vi "SSC DCPower Measure.vi"(0 "DCPower SSC in":T2[](array[typedef]), 5 "Measurement Mode":T1 caption="Measurement Mode (Auto)", 11 "error in":errorcluster) -> (4 "DCPower SSC out":T2[](array[typedef]), 6 "Voltage Measurements (V)":dbl[](array[numeric]) format="%#_6p", 8 "Current Measurements (A)":dbl[](array[numeric]) format="%#_6p", 15 "error out":errorcluster)   [LabVIEW 2020]
doc: "This VI takes a Voltage and Current measurement for each session.\n\nMeasurement Mode is a recommended input. The Auto setting will check the measurement mode for each session and use the appropriate measurement method per session."
uses:
  SSC DCPower.ctl
  Measure/SSC DCPower Measurement Mode.ctl
  <instrlib>/niDCPower/nidcpower.llb/niDCPower Send Software Edge Trigger - Signal.ctl
  Measure/SSC DCPower Debug Global.vi
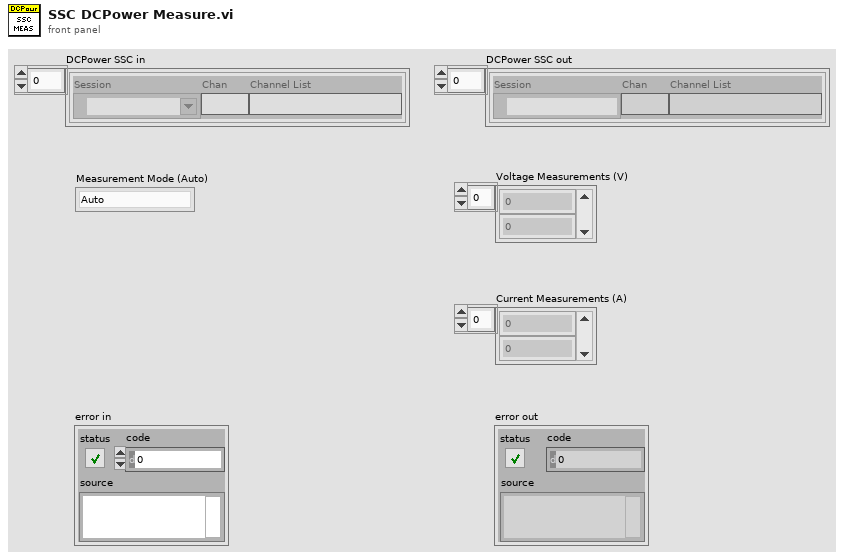
[diagram p1: front panel]
types:
  T1 = typedef "SSC DCPower Measurement Mode.ctl" = enum16{"Auto", "Measure Multiple", "Software Triggers"}
  T2 = typedef "SSC DCPower.ctl" = cluster{"Session":refnum<k15>, "Chan":string, "Channel List":string}
  T3 = typedef "niDCPower Send Software Edge Trigger - Signal.ctl" = i32
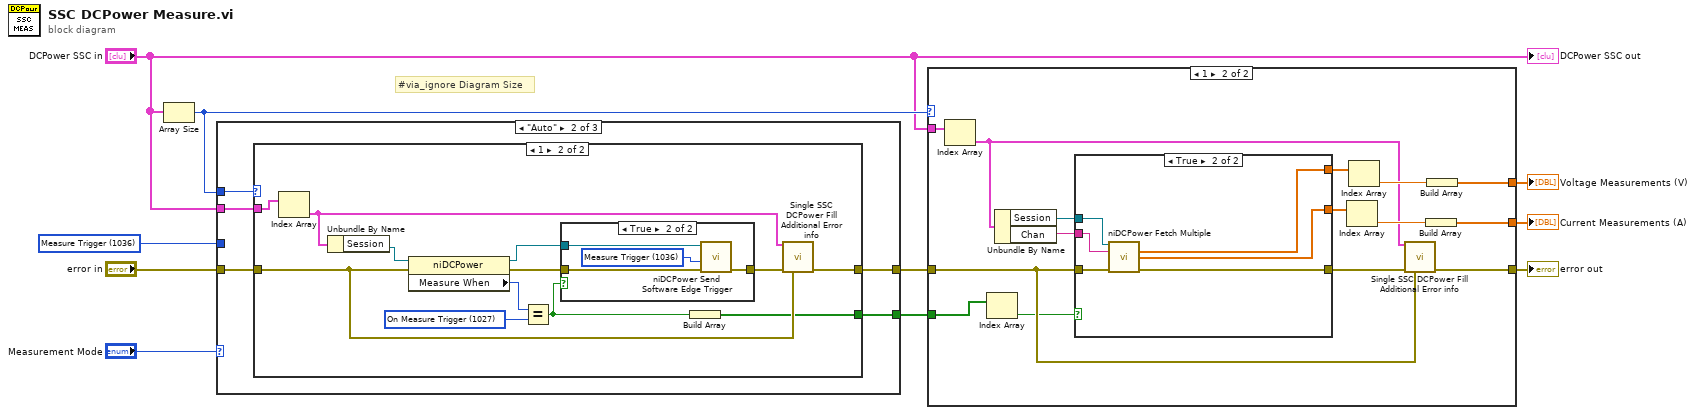
[diagram p0: block diagram]
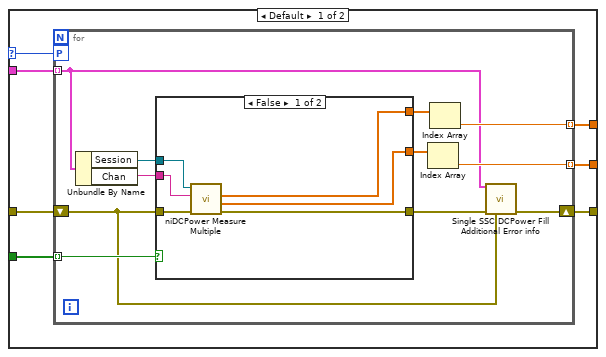
[diagram p2: hidden frame]
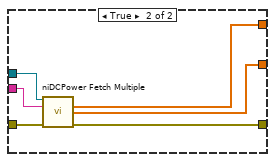
[diagram p3: hidden frame]
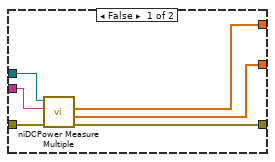
[diagram p4: hidden frame]
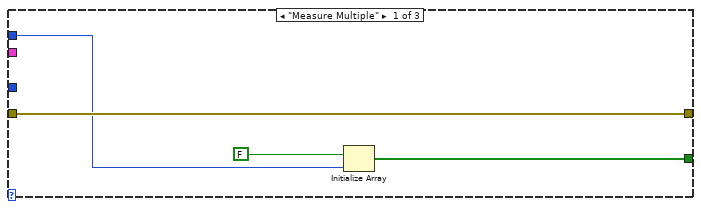
[diagram p5: hidden frame]
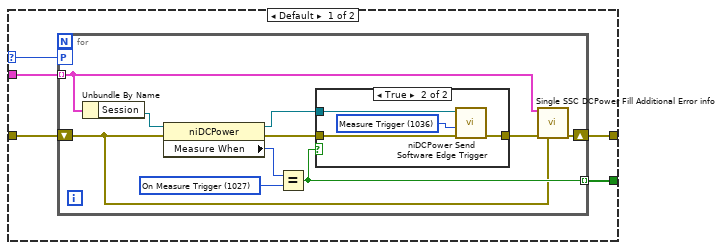
[diagram p6: hidden frame]
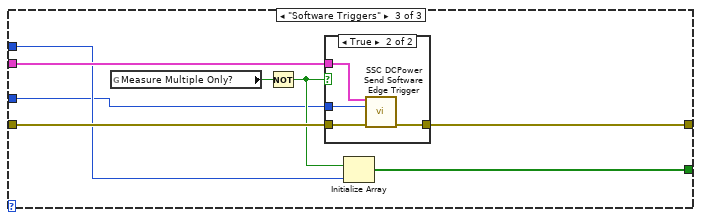
[diagram p9: hidden frame]
diagram:
  w1 = T3 1036 items=["Start Trigger"=1034, "Source Trigger"=1035, "Measure Trigger"=1036, "Sequence Advance Trigger"=1037, "Pulse Trigger"=1053] ("Trigger to Send")
  # "#via_ignore Diagram Size"
  n1 = Array Size(array="DCPower SSC in") -> (size(s)=w7:i32)
  n2 = case shown="\"Auto\"" "Measurement Mode" {
    tunnel: "error in" -> [w14 w19 w64]
    tunnel: [w14 w18 w63] -> w9
    tunnel: w7 -> [w13 w17 w59]
    tunnel: "DCPower SSC in" -> [_ w16 w62]
    tunnel: [w11 w15 w58] -> w3
    tunnel: w1 -> [_ _ w57]
    frame "Measure Multiple" {
      n3 = Initialize Array(FALSE, w13) -> (w11:bool[])
    }
    frame "Auto" {
      n4 = case shown="1" w17 {
        selector: w17 -> [w22 _]
        tunnel: w19 -> [w24 w51]
        tunnel: [w23 w50] -> w18
        tunnel: w16 -> [w21 w49]
        tunnel: [w20 w40] -> w15
        frame Default {
          n5 = for {
            shift-right: [w27] -> w23
            shift-left: w24 -> [w25]
            tunnel: w21 -> [w26] mode=indexing
            workers-P: w22 -> [_]
            tunnel: [w28] -> w20 mode=indexing
            w29 = 1027 items=["Automatically after Source Complete"=1025, "On Demand"=1026, "On Measure Trigger"=1027] ("Measurement:Advanced:Measure When")
            n6 = Unbundle By Name(w26) -> ("Session"=w33:refnum<k15>)
            n7 = property class="niDCPower"(reference=w33, error in=w25) -> (reference out=w31:refnum<k15>, error out=w34:errorcluster, "Measure When"=w30:i32)
            n8 = Equal?(x=w30, y=w29) -> (x = y?=w28:bool)
            n9 = case shown="True" w28 {
              tunnel: w34 -> [w35 w39]
              tunnel: [w35 w38] -> w32
              tunnel: w31 -> [_ w37]
              frame False {
              }
              frame True {
                w36 = T3 1036 items=["Start Trigger"=1034, "Source Trigger"=1035, "Measure Trigger"=1036, "Sequence Advance Trigger"=1037, "Pulse Trigger"=1053] ("signal")
                n10 = call <instrlib>:"niDCPower Send Software Edge Trigger.vi"("error in (no error)"=w39, "signal"=w36, "instrument handle"=w37) -> ("error out"=w38:errorcluster)  [unwired: 7 in, 1 out]
              }
            }
            n11 = call "Single SSC DCPower Fill Additional Error info.vi"("DCPower SSC in"=w26, "error in"=w32, "previous error in"=w25) -> ("error out"=w27:errorcluster)  [unwired: 12 in]
          }
        }
        frame 1 {
          w42 = 1027 items=["Automatically after Source Complete"=1025, "On Demand"=1026, "On Measure Trigger"=1027] ("Measurement:Advanced:Measure When")
          n12 = Index Array(array=w49) -> (element=w41:T2)  [unwired: 1 in]
          n13 = Unbundle By Name(w41) -> ("Session"=w46:refnum<k15>)
          n14 = property class="niDCPower"(reference=w46, error in=w51) -> (reference out=w44:refnum<k15>, error out=w47:errorcluster, "Measure When"=w43:i32)
          n15 = Equal?(x=w43, y=w42) -> (x = y?=w48:bool)
          n16 = case shown="True" w48 {
            tunnel: w47 -> [w52 w56]
            tunnel: [w52 w55] -> w45
            tunnel: w44 -> [_ w54]
            frame False {
            }
            frame True {
              w53 = T3 1036 items=["Start Trigger"=1034, "Source Trigger"=1035, "Measure Trigger"=1036, "Sequence Advance Trigger"=1037, "Pulse Trigger"=1053] ("signal")
              n17 = call <instrlib>:"niDCPower Send Software Edge Trigger.vi"("error in (no error)"=w56, "signal"=w53, "instrument handle"=w54) -> ("error out"=w55:errorcluster)  [unwired: 7 in, 1 out]
            }
          }
          n18 = Build Array(w48) -> (w40:bool[])
          n19 = call "Single SSC DCPower Fill Additional Error info.vi"("DCPower SSC in"=w41, "error in"=w45, "previous error in"=w51) -> ("error out"=w50:errorcluster)  [unwired: 12 in]
        }
      }
    }
    frame "Software Triggers" {
      n20 = global read "SSC DCPower Debug Global.vi" "Measure Multiple Only?"() -> (w61:bool)
      n21 = Not(x=w61) -> (.not. x?=w60:bool)
      n22 = case shown="True" w60 {
        tunnel: w64 -> [w65 w69]
        tunnel: [w65 w68] -> w63
        tunnel: w62 -> [_ w67]
        tunnel: w57 -> [_ w66]
        frame False {
        }
        frame True {
          n23 = call "SSC DCPower Send Software Edge Trigger.vi"("DCPower SSC in"=w67, "Trigger to Send"=w66, "error in"=w69) -> ("error out"=w68:errorcluster)  [unwired: 11 in, 1 out]
        }
      }
      n24 = Initialize Array(w60, w59) -> (w58:bool[])
    }
  }
  n25 = case shown="1" w7 {
    selector: w7 -> [w74 _]
    tunnel: w9 -> [w76 w114]
    tunnel: [w75 w113] -> w8
    tunnel: "DCPower SSC in" -> [w73 w112]
    tunnel: [w72 w101] -> w5
    tunnel: [w71 w100] -> w4
    tunnel: w3 -> [w70 w109]
    frame Default {
      n26 = for {
        shift-right: [w79] -> w75
        shift-left: w76 -> [w77]
        workers-P: w74 -> [_]
        tunnel: w73 -> [w78] mode=indexing
        tunnel: [w82] -> w72 mode=indexing
        tunnel: [w80] -> w71 mode=indexing
        tunnel: w70 -> [w84] mode=indexing
        n27 = Unbundle By Name(w78) -> ("Session"=w86:refnum<k15>, "Chan"=w85:string)
        n28 = case shown="False" w84 {
          tunnel: w77 -> [w93 w99]
          tunnel: [w92 w98] -> w87
          tunnel: w86 -> [w91 w97]
          tunnel: w85 -> [w90 w95]
          tunnel: [w89 w96] -> w83
          tunnel: [w88 w94] -> w81
          frame False {
            n29 = call <instrlib>:"niDCPower Measure Multiple.vi"("error in (no error)"=w93, "channel name"=w90, "instrument handle"=w91) -> ("error out"=w92:errorcluster, "current measurements"=w88:dbl[], "voltage measurements"=w89:dbl[])  [unwired: 5 in, 1 out]
          }
          frame True {
            n30 = call <instrlib>:"niDCPower Fetch Multiple.vi"("instrument handle"=w97, "channel name"=w95, "error in (no error)"=w99) -> ("voltage measurements"=w96:dbl[], "current measurements"=w94:dbl[], "error out"=w98:errorcluster)  [unwired: 7 in, 3 out]
          }
        }
        n31 = Index Array(array=w81) -> (element=w80:dbl)  [unwired: 1 in]
        n32 = Index Array(array=w83) -> (element=w82:dbl)  [unwired: 1 in]
        n33 = call "Single SSC DCPower Fill Additional Error info.vi"("DCPower SSC in"=w78, "error in"=w87, "previous error in"=w77) -> ("error out"=w79:errorcluster)  [unwired: 12 in]
      }
    }
    frame 1 {
      n34 = Index Array(array=w112) -> (element=w103:T2)  [unwired: 1 in]
      n35 = Index Array(array=w109) -> (element=w102:bool)  [unwired: 1 in]
      n36 = Unbundle By Name(w103) -> ("Session"=w107:refnum<k15>, "Chan"=w106:string)
      n37 = case shown="True" w102 {
        tunnel: w114 -> [w120 w126]
        tunnel: [w119 w125] -> w108
        tunnel: w107 -> [w118 w124]
        tunnel: w106 -> [w117 w122]
        tunnel: [w116 w123] -> w105
        tunnel: [w115 w121] -> w104
        frame False {
          n38 = call <instrlib>:"niDCPower Measure Multiple.vi"("error in (no error)"=w120, "channel name"=w117, "instrument handle"=w118) -> ("error out"=w119:errorcluster, "current measurements"=w115:dbl[], "voltage measurements"=w116:dbl[])  [unwired: 5 in, 1 out]
        }
        frame True {
          n39 = call <instrlib>:"niDCPower Fetch Multiple.vi"("instrument handle"=w124, "channel name"=w122, "error in (no error)"=w126) -> ("voltage measurements"=w123:dbl[], "current measurements"=w121:dbl[], "error out"=w125:errorcluster)  [unwired: 7 in, 3 out]
        }
      }
      n40 = Index Array(array=w104) -> (element=w110:dbl)  [unwired: 1 in]
      n41 = Index Array(array=w105) -> (element=w111:dbl)  [unwired: 1 in]
      n42 = call "Single SSC DCPower Fill Additional Error info.vi"("DCPower SSC in"=w103, "error in"=w108, "previous error in"=w114) -> ("error out"=w113:errorcluster)  [unwired: 12 in]
      n43 = Build Array(w110) -> (w100:dbl[])
      n44 = Build Array(w111) -> (w101:dbl[])
    }
  }
  "error out" <- w8
  "Voltage Measurements (V)" <- w5
  "Current Measurements (A)" <- w4
  "DCPower SSC out" <- "DCPower SSC in"
